vi "单控制器监视界面.vi"() -> ()   [LabVIEW 2010]
panel:
  in  "进入配置界面 2":bool
  in  "显示湿度曲线":bool
  in  "显示温度曲线":bool
  in  "选择试验剖面并执行":bool
  in  "试验剖面设置":bool
  in  "单点设置":bool
  in  "退出":bool
  in  "进入配置界面":bool
  in  "当前连接的控制器":string
  out "湿度":dbl
  out "温度":dbl
  out "实测曲线":dbl[](graph)
  # "输出控制量全部off"
  # "当前温度"
  # "当前湿度"
  # "实时曲线显示"
  # "显示当前连接的控制器信息"
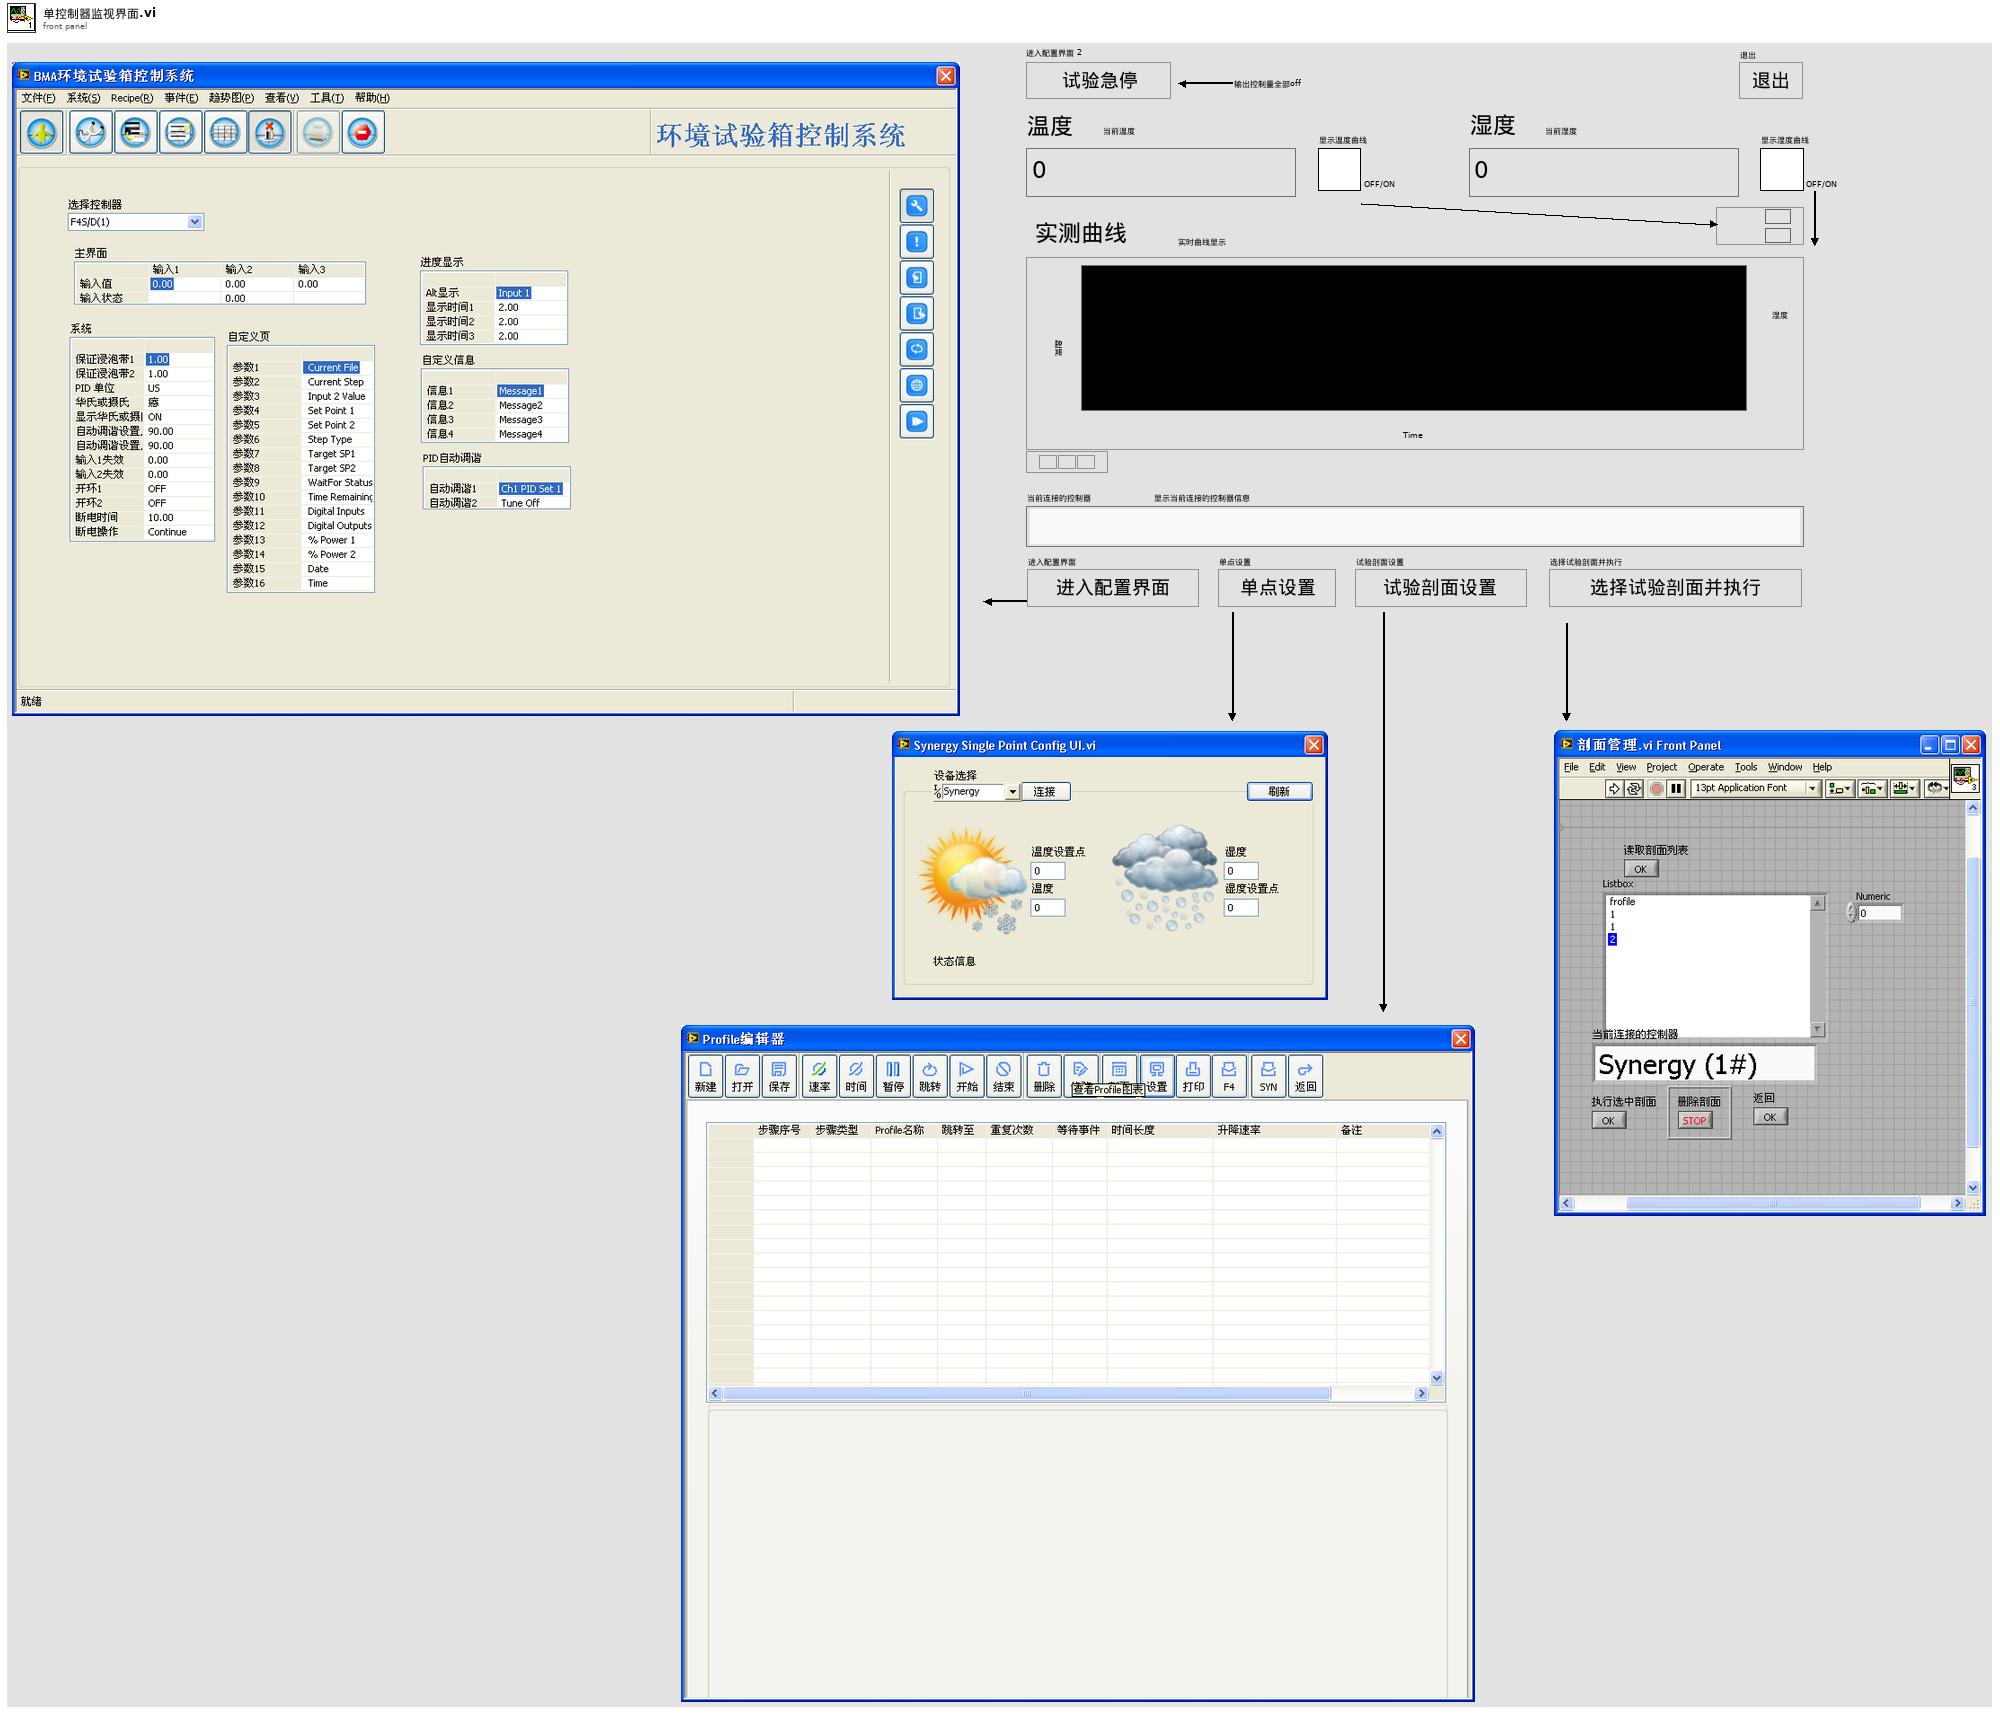
[diagram p1: front panel]
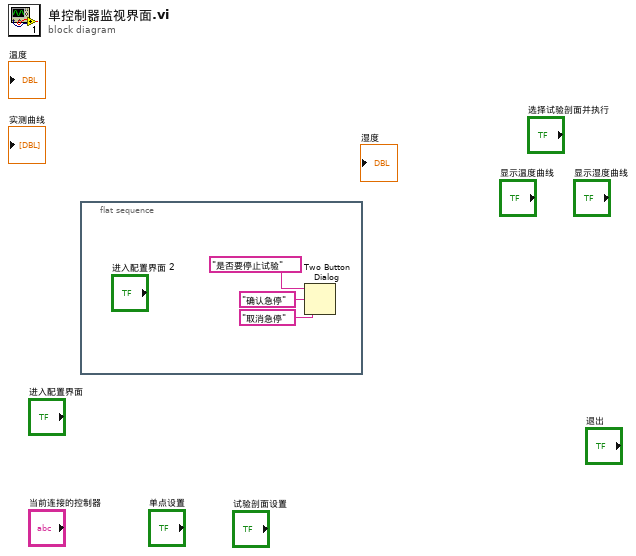
[diagram p0: block diagram]
diagram:
  n1 = flat-sequence {
    frame #0 {
      n2 = Two Button Dialog(message="是否要停止试验", 1:"取消急停" ("F button name (\"Cancel\")"), 2:"确认急停" ("T button name (\"OK\")")) -> ()  [unwired: 1 out]
    }
  }
